vi "3_4_(1).vi"() -> ()   [LabVIEW 2012]
uses:
  Control 1.ctl
panel:
  in  "Відправити серверу":bool
  in  "Відправити клієнту":bool
  in  "Клієнт":string
  in  "Сервер":string
  out "Відповіді":string
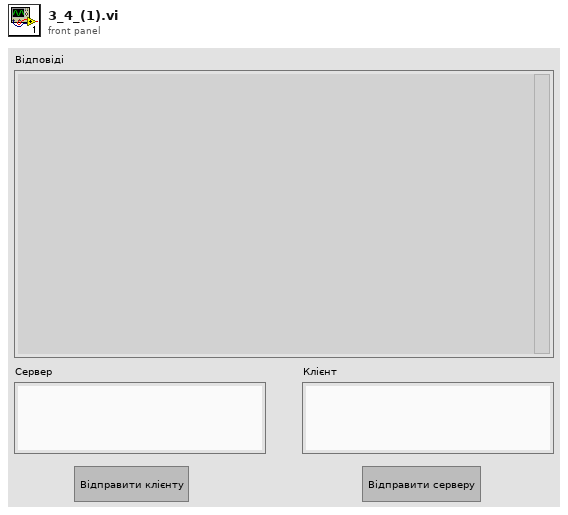
[diagram p1: front panel]
types:
  T1 = cluster{"Відповідь":string, "Enter":string, "Хто":string}
  T2 = typedef "Control 1.ctl" = enum16{"Серверу", "Клієнту", "Зчитати", "Стоп", "1", "2", "3", "4"}
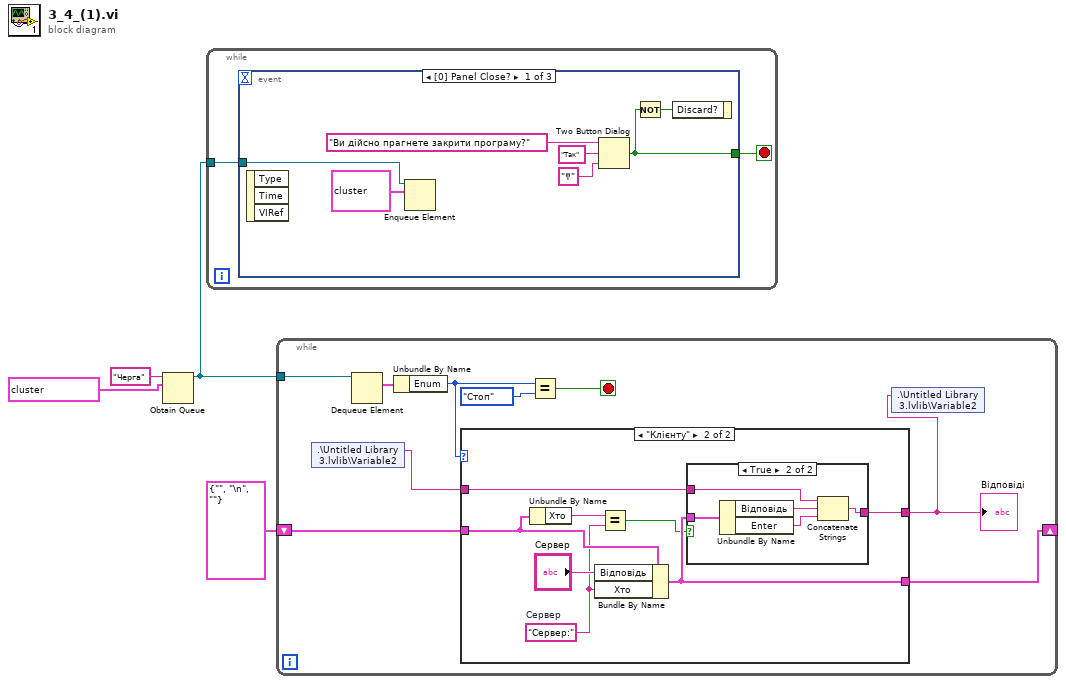
[diagram p0: block diagram]
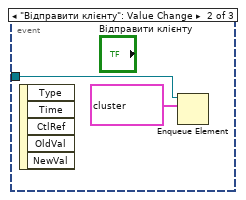
[diagram p2: hidden frame]
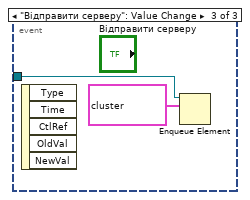
[diagram p3: hidden frame]
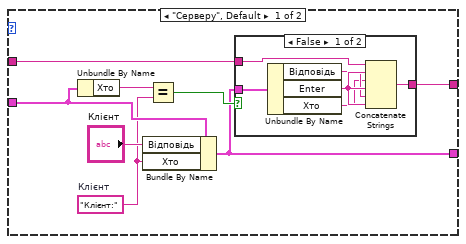
[diagram p4: hidden frame]
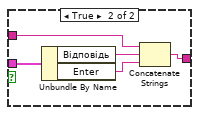
[diagram p5: hidden frame]
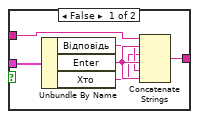
[diagram p6: hidden frame]
diagram:
  n1 = Obtain Queue(name (unnamed)="Черга", element data type=cluster{"variant":variant, "Enum":T2} {"variant"=variant, "Enum"=enum."Стоп"}) -> (queue out=w2:refnum<queue>)  [unwired: 3 in, 2 out]
  n2 = while {
    tunnel: w2 -> [w5]
    stop <- w6 stop-if-true
    n3 = event shown="[0] Panel Close?" {
      selector: _ -> [_ _ _]
      dyn-events: _ -> [_ _ _]
      timeout: _ -> [_ _ _]
      tunnel: [w9 _ _] -> w6
      tunnel: w5 -> [w8 w14 w16]
      event Panel Close? {
        n4 = event-data() -> ()  [unwired: 1 in, 3 out]
        n5 = Enqueue Element(queue=w8, element=cluster{"variant":variant, "Enum":T2} {"variant"=variant, "Enum"=enum."Стоп"}) -> ()  [unwired: 2 in, 3 out]
        n6 = Two Button Dialog(message="Ви дійсно прагнете закрити програму?", 1:"ͳ" ("F button name (\"Cancel\")"), 2:"Так" ("T button name (\"OK\")")) -> (T button?=w9:bool)
        n7 = Not(x=w9) -> (.not. x?=w10:bool)
        n8 = event-data("Discard?"=w10) -> ()  [unwired: 1 in, 1 out]
      }
      event "Відправити клієнту": Value Change {
        n9 = event-data() -> ()  [unwired: 1 in, 5 out]
        n10 = Enqueue Element(queue=w14, element=cluster{"variant":variant, "Enum":T2} {"variant"=variant, "Enum"=enum."Клієнту"}) -> ()  [unwired: 2 in, 3 out]
      }
      event "Відправити серверу": Value Change {
        n11 = event-data() -> ()  [unwired: 1 in, 5 out]
        n12 = Enqueue Element(queue=w16, element=cluster{"variant":variant, "Enum":T2} {"variant"=variant, "Enum"=enum."Серверу"}) -> ()  [unwired: 2 in, 3 out]
      }
    }
  }
  n13 = while {
    tunnel: w2 -> [w26]
    shift-right: [w20] -> _
    shift-left: T1 {"Відповідь"="", "Enter"="\n", "Хто"=""} -> [w21]
    stop <- w23 stop-if-true
    n14 = shared-variable ".\\Untitled Library 3.lvlib\\Variable2"() -> (w19:string)  [unwired: 1 in, 1 out]
    n15 = Dequeue Element(queue=w26) -> (element=w25:cluster{"variant":variant, "Enum":T2})  [unwired: 2 in, 3 out]
    n16 = Unbundle By Name(w25) -> ("Enum"=w22:T2)
    n17 = case shown="\"Клієнту\"" w22 {
      tunnel: w21 -> [w33 w49]
      tunnel: [w29 w52] -> w20
      tunnel: [w28 w50] -> w18
      tunnel: w19 -> [w27 w51]
      frame "Серверу", Default {
        w31 = "Клієнт:"  # Клієнт
        n18 = Unbundle By Name(w33) -> ("Хто"=w32:string)
        n19 = Bundle By Name(cluster=w33, "Відповідь"="Клієнт", "Хто"=w31) -> (w29:T1)
        n20 = Equal?(x=w32, y=w31) -> (x = y?=w30:bool)
        n21 = case shown="False" w30 {
          tunnel: w29 -> [w37 w45]
          tunnel: [w36 w44] -> w28
          tunnel: w27 -> [w35 w43]
          frame False {
            n22 = Unbundle By Name(w37) -> ("Відповідь"=w39:string, "Enter"=w40:string, "Хто"=w38:string)
            n23 = Concatenate Strings(w35, w40, w38, w40, w39, w40) -> (w36:string)
          }
          frame True {
            n24 = Unbundle By Name(w45) -> ("Відповідь"=w42:string, "Enter"=w41:string)
            n25 = Concatenate Strings(w43, w42, w41) -> (w44:string)
          }
        }
      }
      frame "Клієнту" {
        w47 = "Сервер:"  # Сервер
        n26 = Unbundle By Name(w49) -> ("Хто"=w48:string)
        n27 = Bundle By Name(cluster=w49, "Відповідь"="Сервер", "Хто"=w47) -> (w52:T1)
        n28 = Equal?(x=w48, y=w47) -> (x = y?=w46:bool)
        n29 = case shown="True" w46 {
          tunnel: w52 -> [w56 w64]
          tunnel: [w55 w63] -> w50
          tunnel: w51 -> [w54 w62]
          frame False {
            n30 = Unbundle By Name(w56) -> ("Відповідь"=w58:string, "Enter"=w59:string, "Хто"=w57:string)
            n31 = Concatenate Strings(w54, w59, w57, w59, w58, w59) -> (w55:string)
          }
          frame True {
            n32 = Unbundle By Name(w64) -> ("Відповідь"=w61:string, "Enter"=w60:string)
            n33 = Concatenate Strings(w62, w61, w60) -> (w63:string)
          }
        }
      }
    }
    "Відповіді" <- w18
    n34 = Equal?(x=w22, y=Control_1."Стоп" ("Enum")) -> (x = y?=w23:bool)
    n35 = shared-variable ".\\Untitled Library 3.lvlib\\Variable2"(w18) -> ()  [unwired: 1 in, 1 out]
  }
